vi "channelselectexample.vi"() -> ()   [LabVIEW 2015]
panel:
  out "CI":dbl[](array[numeric])
  out "AI":dbl[](array[numeric])
  in  "AI":i32[](listbox)
  in  "CI":i32[](listbox)
  in  "stop":bool
  out "Array 2":dbl[](array[numeric])
  out "Array":dbl[](array[numeric])
  in  "add DO":bool
  in  "add AO":bool
  in  "DO":u16(ring) items=["2p Shutter", "488 shutter (not in use)", "camera trigger", "640 shutter", "LT timestamp"]
  in  "AO":u16(ring) items=["X", "Y", "Voltage to patch", "CW laser"]
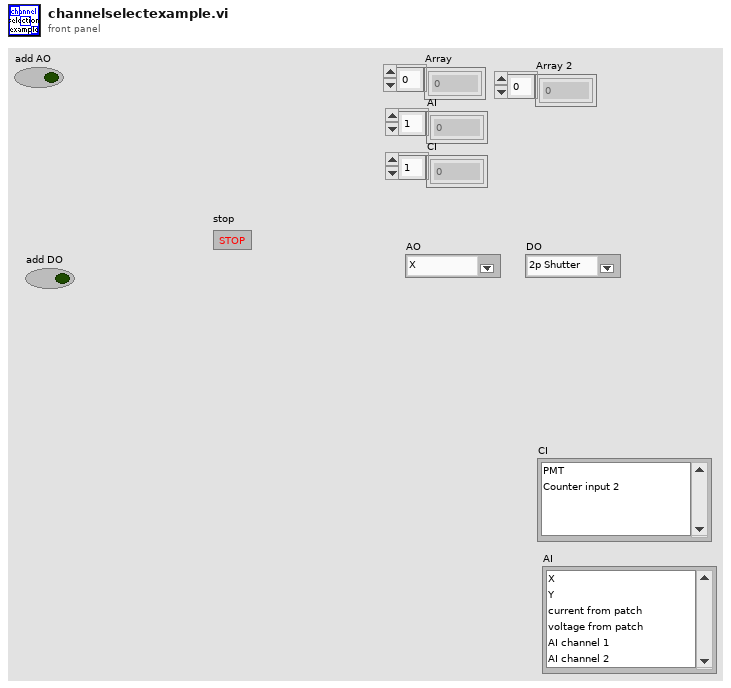
[diagram p1: front panel]
types:
  T1 = typedef "XYZStage.lvlib/XYZStage Configuration.ctl" = cluster{"VISA resource name":refnum<visa-resource-name>, "Timeout (3sec)":u32}
  T2 = cluster{"StageS":i32, "StageL":i32, "currmeas data dir":path, "image OD":u16, "contour OD":u16, "point OD":u16, "AOlines":tag[], "AIlines":tag[], "CI lines":tag[], "DO lines":tag[], "AO names":string[], "CI names":string[], "AI names":string[], "DO names":string[], "CIextensions":string[], "AIextensions":string[], "Voltage to Ygalvo":i32, "Voltage to Xgalvo":i32, "Voltage to patch":i32, "640 shutter":i32, "2P shutter":i32, "LT timestamp":u32, "Vp":i32, "Ip":i32, "camera trigger":i32, "master data dir":path, "voltage to Zpos":i32, "Vto2P":i32, "640 AO":i32, "488 AO":i32, "532 AO":i32, "640TTL":u32, "488TTL":u32, "532TTL":u32, "Device 1 sampleclock out":tag, "Device 1 Starttrigger out":tag, "Device 2 sampleclock in":tag, "Device 2 StartTrigger in ":tag, "2PODTTL":u32, "488 shutter":u32, "LCVR red":u32, "LCVR blue":u32, "Sutter Stage Config":T1}
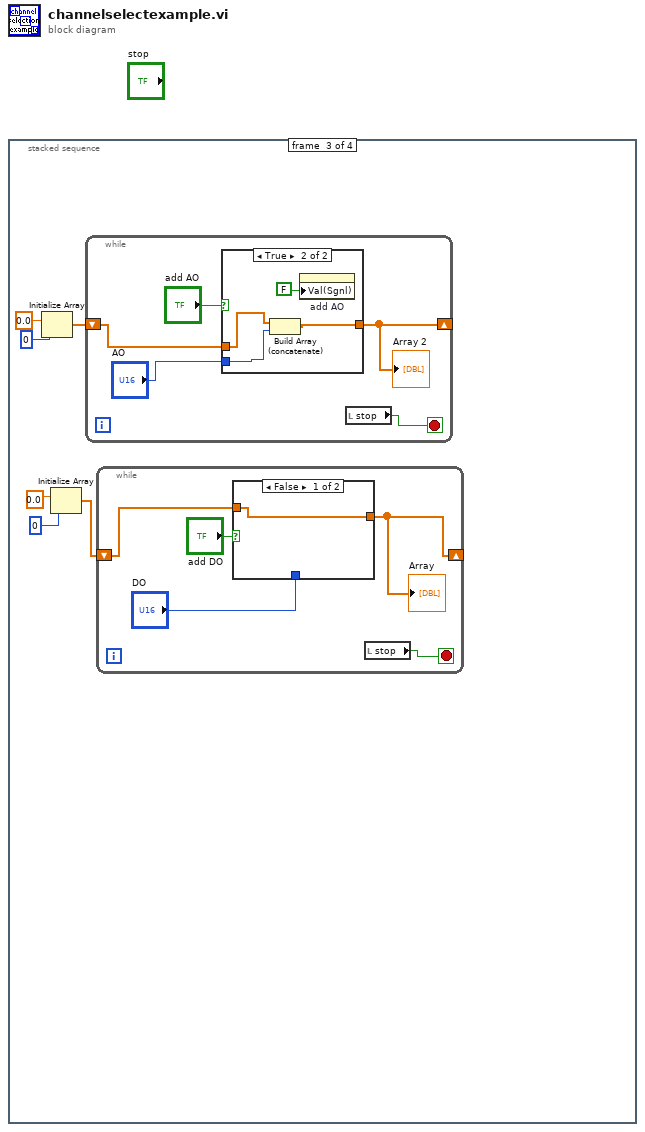
[diagram p0: block diagram]
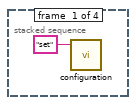
[diagram p2: hidden frame]
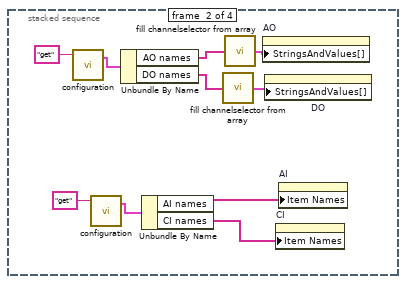
[diagram p3: hidden frame]
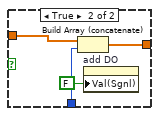
[diagram p4: hidden frame]
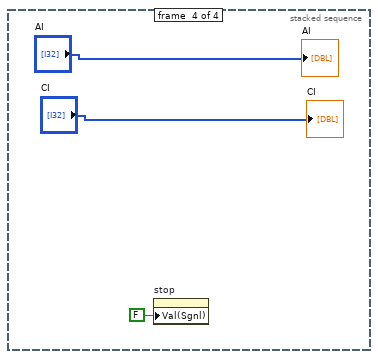
[diagram p6: hidden frame]
diagram:
  n1 = stacked-sequence {
    frame #0 {
      n2 = call "configuration.vi"("command"="set") -> ()  [unwired: 2 in, 2 out]
    }
    frame #1 {
      n3 = call "configuration.vi"("command"="get") -> ("config out"=w11:T2)  [unwired: 2 in, 1 out]
      n4 = call "configuration.vi"("command"="get") -> ("config out"=w4:T2)  [unwired: 2 in, 1 out]
      n5 = Unbundle By Name(w11) -> ("AO names"=w9:string[], "DO names"=w8:string[])
      n6 = Unbundle By Name(w4) -> ("AI names"=w3:string[], "CI names"=w2:string[])
      n7 = call "fill channelselector from array.vi"("channel  names"=w8) -> ("channel selector string and values"=w6:cluster{"String":string, "Value":u16}[])
      n8 = call "fill channelselector from array.vi"("channel  names"=w9) -> ("channel selector string and values"=w7:cluster{"String":string, "Value":u16}[])
      n9 = property on="AO" class="Ring (strict)"("StringsAndValues[]"=w7) -> ()  [unwired: 2 in, 2 out]
      n10 = property on="DO" class="Ring (strict)"("StringsAndValues[]"=w6) -> ()  [unwired: 2 in, 2 out]
      n11 = property on="CI" class="LstBox (strict)"("Item Names"=w2) -> ()  [unwired: 2 in, 2 out]
      n12 = property on="AI" class="LstBox (strict)"("Item Names"=w3) -> ()  [unwired: 2 in, 2 out]
    }
    frame #2 {
      n13 = Initialize Array(0.0 ("element"), 0 ("dimension size")) -> (w17:dbl[])
      n14 = Initialize Array(0.0 ("element"), 0 ("dimension size")) -> (w12:dbl[])
      n15 = while {
        shift-right: [w28] -> _
        shift-left: w17 -> [w31]
        stop <- w29 stop-if-true
        n16 = case shown="True" "add AO" {
          tunnel: w31 -> [w33 w36]
          tunnel: "AO" -> [_ w35]
          tunnel: [w33 w37] -> w28
          frame False {
          }
          frame True {
            n17 = Build Array (concatenate)(w36, w35) -> (w37:dbl[])
            n18 = property on="add AO" class="Bool (strict)"("Val(Sgnl)"=FALSE) -> ()  [unwired: 2 in, 2 out]
          }
        }
        "Array 2" <- w28
        n19 = local read "stop"() -> (w29:bool)
      }
      n20 = while {
        shift-right: [w18] -> _
        shift-left: w12 -> [w21]
        stop <- w19 stop-if-true
        n21 = case shown="False" "add DO" {
          tunnel: w21 -> [w23 w27]
          tunnel: "DO" -> [_ w26]
          tunnel: [w23 w25] -> w18
          frame False {
          }
          frame True {
            n22 = Build Array (concatenate)(w27, w26) -> (w25:dbl[])
            n23 = property on="add DO" class="Bool (strict)"("Val(Sgnl)"=FALSE ("Value (Signaling)")) -> ()  [unwired: 2 in, 2 out]
          }
        }
        "Array" <- w18
        n24 = local read "stop"() -> (w19:bool)
      }
    }
    frame #3 {
      n25 = property on="stop" class="Bool (strict)"("Val(Sgnl)"=FALSE ("Value (Signaling)")) -> ()  [unwired: 2 in, 2 out]
      "AI" <- "AI"
      "CI" <- "CI"
    }
  }
